vi "Calculation_Angle_Between_Displacements-1.vi"(1 "dY 2":dbl, 2 "dX 2":dbl, 3 "dY 1":dbl, 4 "dX 1":dbl) -> (0 "angle in degrees":dbl)   [LabVIEW 2013]
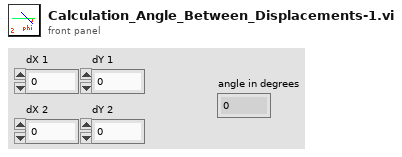
[diagram p1: front panel]
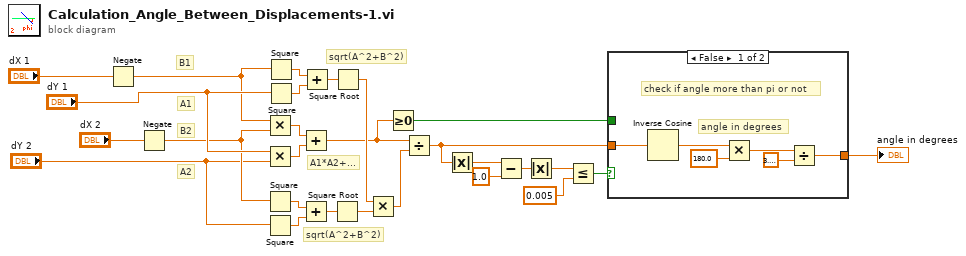
[diagram p0: block diagram]
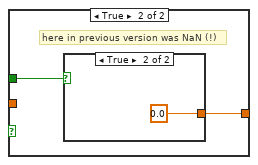
[diagram p2: hidden frame]
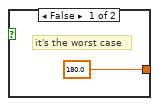
[diagram p3: hidden frame]
diagram:
  # "sqrt(A^2+B^2)"
  # "A1*A2+..."
  # "sqrt(A^2+B^2)"
  # "A2"
  # "B2"
  # "A1"
  # "B1"
  n1 = Negate(x="dX 1") -> (-x=w12:dbl)
  n2 = Negate(x="dX 2") -> (-x=w10:dbl)
  n3 = Multiply(x=w12, y=w10) -> (x*y=w27:dbl)
  n4 = Multiply(x="dY 1", y="dY 2") -> (x*y=w26:dbl)
  n5 = Square(x=w10) -> (x^2=w22:dbl)
  n6 = Square(x="dY 2") -> (x^2=w21:dbl)
  n7 = Square(x=w12) -> (x^2=w25:dbl)
  n8 = Square(x="dY 1") -> (x^2=w24:dbl)
  n9 = Add(x=w27, y=w26) -> (x+y=w16:dbl)
  n10 = Add(x=w22, y=w21) -> (x+y=w20:dbl)
  n11 = Add(x=w25, y=w24) -> (x+y=w23:dbl)
  n12 = Square Root(x=w20) -> (sqrt(x)=w18:dbl)
  n13 = Square Root(x=w23) -> (sqrt(x)=w19:dbl)
  n14 = Multiply(x=w19, y=w18) -> (x*y=w17:dbl)
  n15 = Greater Or Equal To 0?(x=w16) -> (x >= 0?=w15:bool)
  n16 = Divide(x=w16, y=w17) -> (x/y=w2:dbl)
  n17 = Absolute Value(x=w2) -> (abs(x)=w1:dbl)
  n18 = Subtract(x=w1, y=1.0) -> (x-y=w6:dbl)
  n19 = Absolute Value(x=w6) -> (abs(x)=w5:dbl)
  n20 = Less Or Equal?(x=w5, y=0.005) -> (x <= y?=w3:bool)
  n21 = case shown="False" w3 {
    tunnel: w15 -> [_ w34]
    tunnel: [w30 w35] -> w8
    tunnel: w2 -> [w29 _]
    frame False {
      # "check if angle more than pi or not"
      # "angle in degrees"
      n22 = Inverse Cosine(1:w29) -> (0:w28:dbl)
      n23 = Multiply(x=w28, y=180.0) -> (x*y=w32:dbl)
      n24 = Divide(x=w32, y=3.141592653589793) -> (x/y=w30:dbl)
    }
    frame True {
      # "here in previous version was NaN (!)"
      n25 = case shown="True" w34 {
        tunnel: [180.0 0.0] -> w35
        frame False {
          # "it's the worst case"
        }
        frame True {
        }
      }
    }
  }
  "angle in degrees" <- w8
